vi "Pipes_Generate.vi"(7 "Opening Width":dbl=6.0, 8 "error in (no error)":errorcluster, 9 "X&Y-Lower Lim":cluster{sgl[], sgl[]}, 10 "X&Y-Upper Lim":cluster{sgl[], sgl[]}, 11 "Gen Pipe":bool=TRUE) -> (0 "error out":errorcluster, 1 "X&YUpper":cluster{"x":sgl[], "y_upper":sgl[]}, 2 "X&YLower":cluster{"x":sgl[], "y_lower":sgl[]}, 4 "Lower Limit":dbl, 5 "Upper Limit":dbl)   [LabVIEW 2017, in "Flappy Bird.lvlib"]
uses:
  Flappy Bird.lvlib
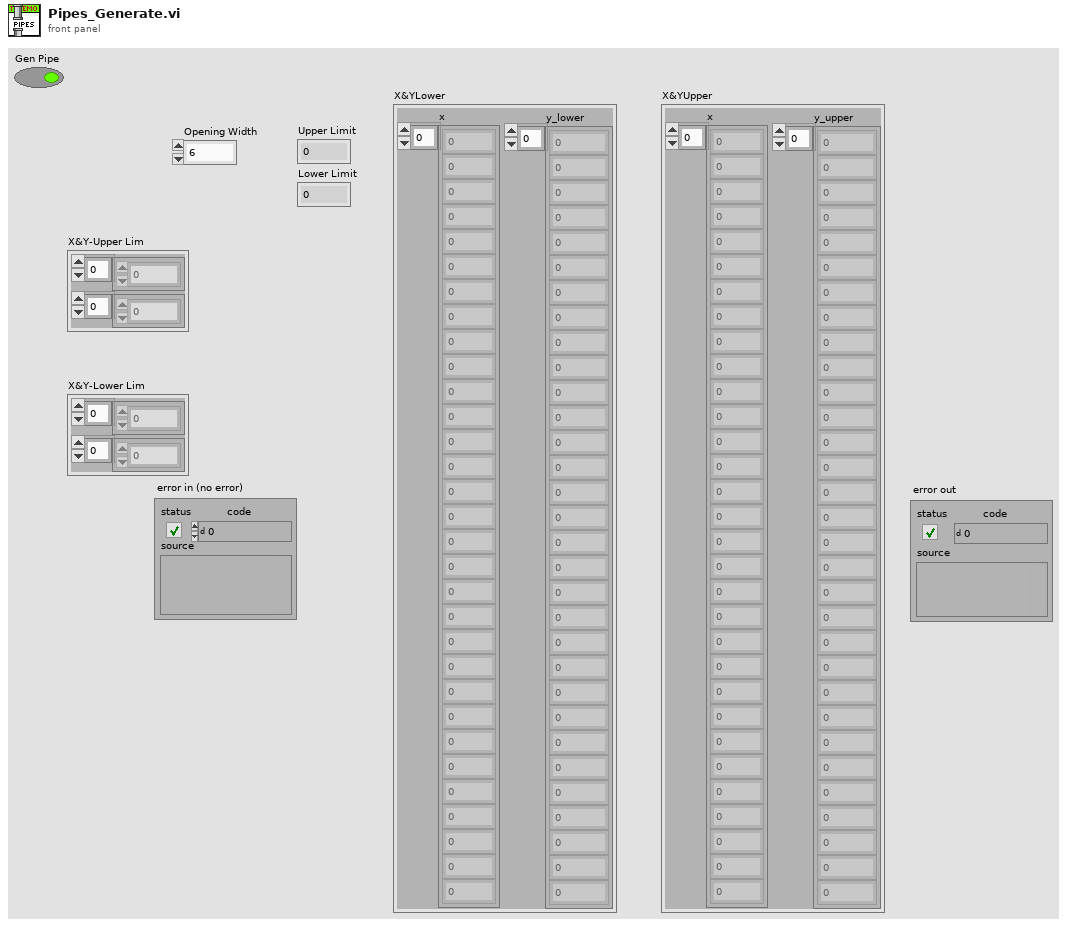
[diagram p1: front panel]
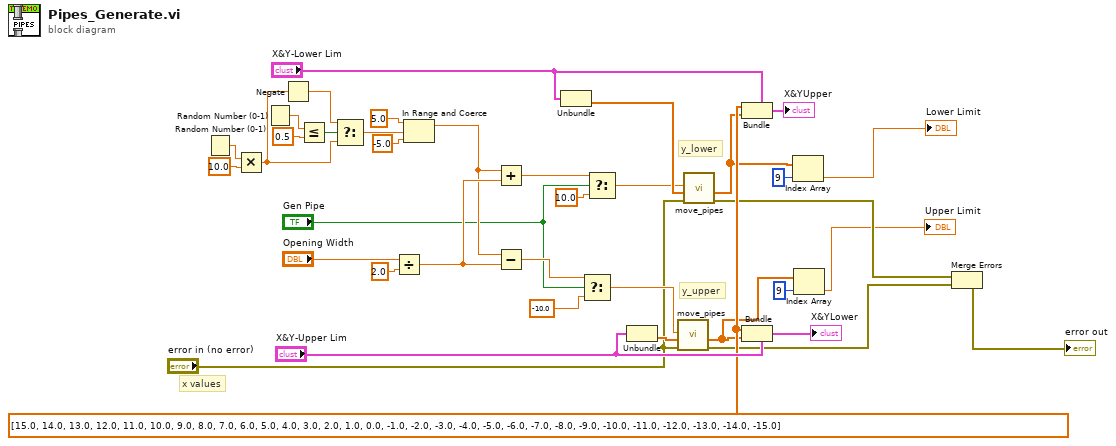
[diagram p0: block diagram]
diagram:
  w14 = sgl[] [15.0, 14.0, 13.0, 12.0, 11.0, 10.0, 9.0, 8.0, 7.0, 6.0, 5.0, 4.0, 3.0, 2.0, 1.0, 0.0, -1.0, -2.0, -3.0, -4.0, -5.0, -6.0, -7.0, -8.0, -9.0, -10.0, -11.0, -12.0, -13.0, -14.0, -15.0]
  # "x values"
  # "y_upper"
  # "y_lower"
  n1 = Random Number (0-1)() -> (number: 0 to 1=w33:dbl)
  n2 = Multiply(x=w33, y=10.0) -> (x*y=w22:dbl)
  n3 = Random Number (0-1)() -> (number: 0 to 1=w25:dbl)
  n4 = Negate(x=w22) -> (-x=w21:dbl)
  n5 = Less Or Equal?(x=w25, y=0.5 ("x")) -> (x <= y?=w23:bool)
  n6 = Select(t=w21, s=w23, f=w22) -> (s? t:f=w20:dbl)
  n7 = Divide(x="Opening Width", y=2.0) -> (x/y=w28:dbl)
  n8 = In Range and Coerce(upper limit=5.0, x=w20, lower limit=-5.0) -> (coerced(x)=w27:dbl)  [unwired: 1 out]
  n9 = Add(x=w27, y=w28) -> (x+y=w19:dbl)
  n10 = Subtract(x=w27, y=w28) -> (x-y=w26:dbl)
  n11 = Unbundle("X&Y-Lower Lim") -> (w16:sgl[])  [unwired: 1 out]
  n12 = Select(t=w26, s="Gen Pipe", f=-10.0 ("t")) -> (s? t:f=w12:dbl)
  n13 = Select(t=w19, s="Gen Pipe", f=10.0) -> (s? t:f=w13:dbl)
  n14 = Unbundle("X&Y-Upper Lim") -> (w15:sgl[])  [unwired: 1 out]
  n15 = call "move_pipes.vi"("error in (no error)"="error in (no error)", "Y-values"=w15, "New Y-value"=w12) -> ("error out"=w8:errorcluster, "Y-values Out"=w6:dbl[])  [unwired: 7 in]
  n16 = call "move_pipes.vi"("error in (no error)"="error in (no error)", "Y-values"=w16, "New Y-value"=w13) -> ("error out"=w9:errorcluster, "Y-values Out"=w3:dbl[])  [unwired: 7 in]
  n17 = Bundle(cluster="X&Y-Lower Lim", w14, w3) -> (→"X&YUpper":cluster{sgl[], sgl[]})
  n18 = Bundle(cluster="X&Y-Upper Lim", w14, w6) -> (→"X&YLower":cluster{sgl[], sgl[]})
  n19 = Index Array(array=w3, index=9) -> (element=→"Lower Limit":dbl)
  n20 = Index Array(array=w6, index=9) -> (element=→"Upper Limit":dbl)
  n21 = Merge Errors(w9, w8) -> (→"error out":errorcluster)
